vi "transform.vi"(0 "GenericTrajectory in":refnum<class "TrajectoryDL091126GenericVoxel.lvclass">, 1 "block size":i32=100000, 2 "number of pixels (all: -1)":i32=-1, 5 "transformation parameters":T1={"scale factor"=1.0, "rotation angle"=0.0, "tilting angle"=0.0, "offset"=refnum}, 11 "error in (no error)":errorcluster) -> (4 "GenericTrajectory out":refnum<class "TrajectoryDL091126GenericVoxel.lvclass">, 6 "x coordinates":dbl[unit][](array[numeric]), 8 "y coordinates":dbl[unit][](array[numeric]), 10 "z coordinates":dbl[unit][](array[numeric]), 15 "error out":errorcluster)   [LabVIEW 2010, in "TrajectoryDL091126GenericVoxel.lvclass"]
uses:
  TrajectoryDL091126GenericVoxel.lvclass
  transformation_parameters.ctl
  common/classes/SpaceVector/SpaceVector/SpaceVector.lvclass
  common/enumerations/x_y_z_enumeration.ctl
  common/enumerations/functional_global_action_enum.ctl
  TrajectoryDL091126GenericVoxel.lvclass/TrajectoryDL091126GenericVoxel.ctl
  <vilib>/Analysis/Matrix/Numeric/Conversions/Array To Matrix - RA2.vi
  <vilib>/Analysis/baseanly.llb/Real A x B.vi
  <vilib>/Analysis/Matrix/Numeric/Conversions/Matrix To Array - RM.vi
  common/classes/ErrorController/ErrorController/class_data.vi
  <vilib>/Analysis/Matrix/NI_Matrix.lvlib
  <vilib>/Analysis/NI_AALBase.lvlib
  common/classes/ErrorController/ErrorController/ErrorController.lvclass
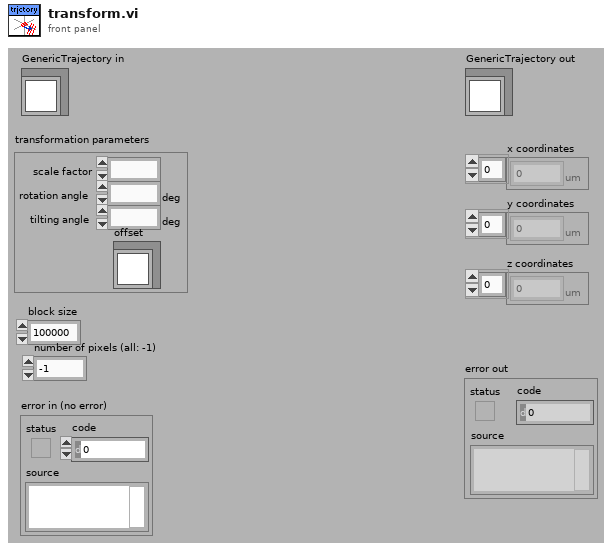
[diagram p1: front panel]
types:
  T1 = typedef "TrajectoryDL091126GenericVoxel.lvclass/transformation_parameters.ctl" = cluster{"scale factor":dbl, "rotation angle":dbl[unit], "tilting angle":dbl[unit], "offset":refnum<class "SpaceVector.lvclass">}
  T2 = typedef "x_y_z_enumeration.ctl" = enum16{"x", "y", "z"}
  T3 = typedef "functional_global_action_enum.ctl" = enum16{"get", "set", "reset"}
  T4 = typedef "NI_Matrix.lvlib/RealMatrix.ctl" = dbl[][]
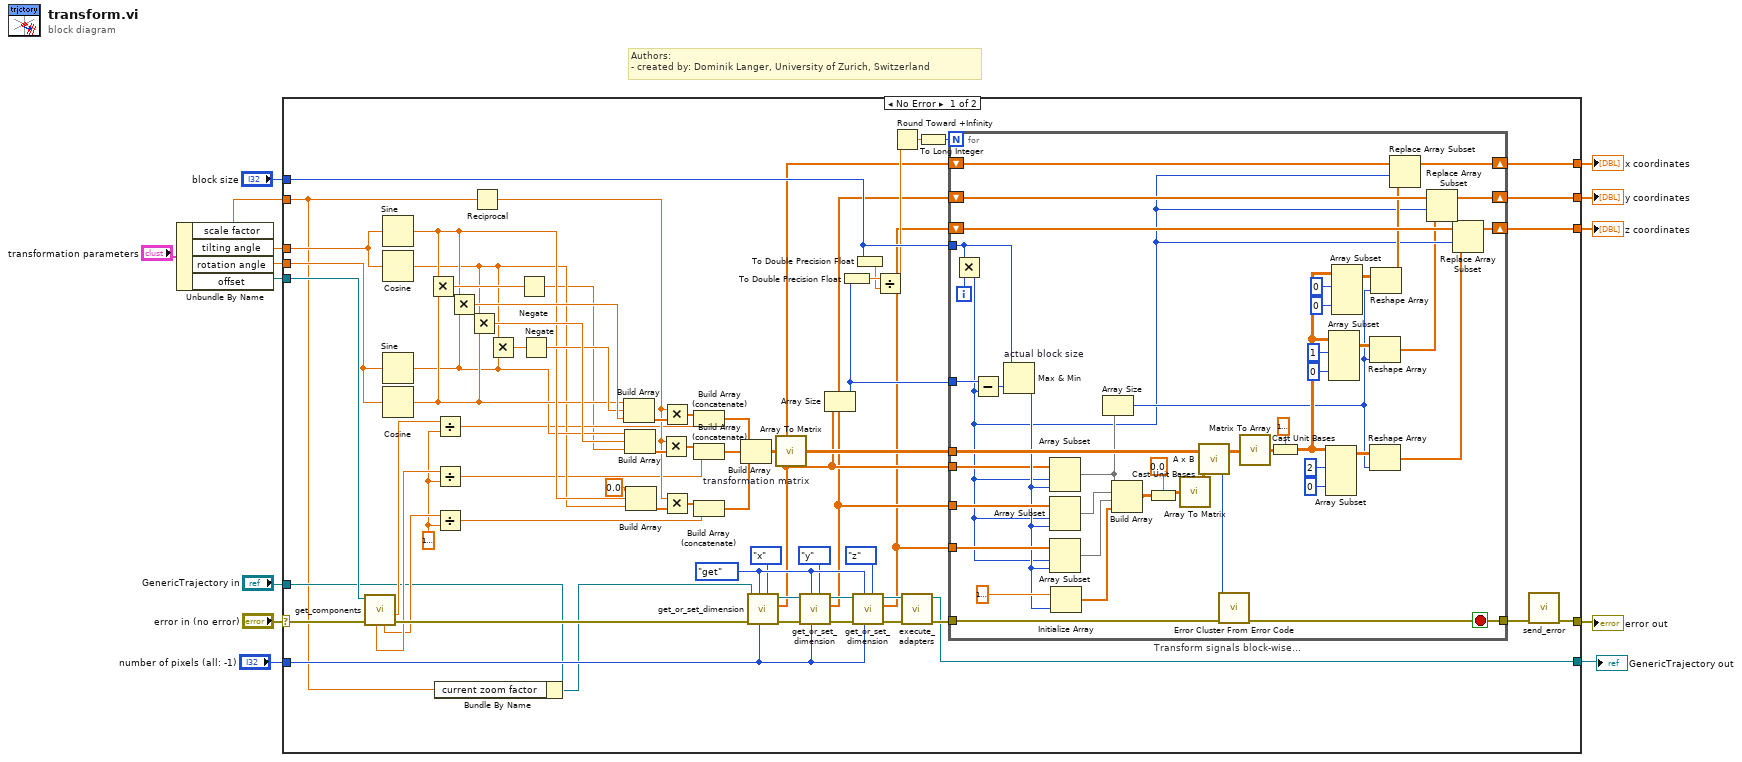
[diagram p0: block diagram]
diagram:
  # "Authors: \n- created by: Dominik Langer, University of Zurich, Switzerland"
  n1 = Unbundle By Name("transformation parameters") -> ("scale factor"=w8:dbl, "tilting angle"=w7:dbl[unit], "rotation angle"=w6:dbl[unit], "offset"=w5:refnum<class "SpaceVector.lvclass">)
  n2 = case shown="No Error" "error in (no error)" {
    selector: "error in (no error)" -> [w66 w127]
    tunnel: [w22 w127] -> w13
    tunnel: [w38 w126] -> w11
    tunnel: "GenericTrajectory in" -> [w18 w126]
    tunnel: w5 -> [w64 _]
    tunnel: w7 -> [w63 _]
    tunnel: w8 -> [w16 _]
    tunnel: "block size" -> [w51 _]
    tunnel: w6 -> [w53 _]
    tunnel: [w49 _] -> w4
    tunnel: [w48 _] -> w3
    tunnel: [w47 _] -> w2
    tunnel: "number of pixels (all: -1)" -> [w24 _]
    frame No Error {
      w34 = dbl[unit] 1e-06 ("unit (none)")
      w78 = functional_global_action_enum."get" ("action")
      n3 = call "get_components.vi"("error in (no error)"=w66, "SpaceVector in"=w64) -> ("error out"=w65:errorcluster, "x"=w37:dbl[unit], "z"=w35:dbl[unit], "y"=w36:dbl[unit])  [unwired: 4 in, 2 out]
      n4 = Sine(x=w63) -> (sin(x)=w62:dbl)
      n5 = Cosine(x=w63) -> (cos(x)=w59:dbl)
      n6 = Sine(x=w53) -> (sin(x)=w60:dbl)
      n7 = Cosine(x=w53) -> (cos(x)=w61:dbl)
      n8 = Multiply(x=w62, y=w61) -> (x*y=w71:dbl)
      n9 = Divide(x=w37, y=w34) -> (x/y=w32:dbl)
      n10 = Divide(x=w36, y=w34) -> (x/y=w28:dbl)
      n11 = Divide(x=w35, y=w34) -> (x/y=w27:dbl)
      n12 = Bundle By Name(cluster=w18, "current zoom factor"=w16) -> (w17:refnum<class "TrajectoryDL091126GenericVoxel.lvclass">)
      n13 = Multiply(x=w62, y=w60) -> (x*y=w69:dbl)
      n14 = Multiply(x=w59, y=w61) -> (x*y=w70:dbl)
      n15 = Reciprocal(x=w16) -> (1/x=w42:dbl)
      n16 = Multiply(x=w59, y=w60) -> (x*y=w67:dbl)
      n17 = Negate(x=w71) -> (-x=w15:dbl)
      n18 = Negate(x=w67) -> (-x=w68:dbl)
      n19 = Build Array(w61, w68, w69) -> (w56:dbl[])
      n20 = Build Array(w60, w70, w15) -> (w55:dbl[])
      n21 = Build Array(0.0, w62, w59) -> (w54:dbl[])
      n22 = Multiply(x=w42, y=w55) -> (x*y=w30:dbl[])
      n23 = Multiply(x=w42, y=w56) -> (x*y=w33:dbl[])
      n24 = Multiply(x=w42, y=w54) -> (x*y=w29:dbl[])
      n25 = Build Array (concatenate)(w33, w32) -> (w31:dbl[])
      n26 = Build Array (concatenate)(w30, w28) -> (w26:dbl[])
      n27 = Build Array (concatenate)(w29, w27) -> (w25:dbl[])
      n28 = Build Array "transformation matrix"(w31, w26, w25) -> (w57:dbl[][])
      n29 = call-dynamic "get_or_set_dimension.vi"("dimension"=x_y_z_enumeration."x", "number of pixels to get (-1: get all)"=w24, "action"=w78, "error in (no error)"=w65, "GenericTrajectory in"=w17) -> ("error out"=w80:errorcluster, "pixel values out (single dimension)"=w21:dbl[unit][], "GenericTrajectory out"=w74:refnum<class "TrajectoryDL091126GenericVoxel.lvclass">)  [unwired: 4 in]
      n30 = call-poly <vilib>:"Array To Matrix.vi"("Real 2D Array"=w57) -> ("Real Matrix"=w58:T4)
      n31 = call-dynamic "get_or_set_dimension.vi"("dimension"=x_y_z_enumeration."y", "number of pixels to get (-1: get all)"=w24, "action"=w78, "error in (no error)"=w80, "GenericTrajectory in"=w74) -> ("error out"=w79:errorcluster, "pixel values out (single dimension)"=w20:dbl[unit][], "GenericTrajectory out"=w73:refnum<class "TrajectoryDL091126GenericVoxel.lvclass">)  [unwired: 4 in]
      n32 = Array Size(array=w21) -> (size(s)=w46:i32)
      n33 = To Double Precision Float(number=w46) -> (double precision float=w52:dbl)
      n34 = call-dynamic "get_or_set_dimension.vi"("dimension"=x_y_z_enumeration."z", "number of pixels to get (-1: get all)"=w24, "action"=w78, "error in (no error)"=w79, "GenericTrajectory in"=w73) -> ("error out"=w41:errorcluster, "pixel values out (single dimension)"=w19:dbl[unit][], "GenericTrajectory out"=w39:refnum<class "TrajectoryDL091126GenericVoxel.lvclass">)  [unwired: 4 in]
      n35 = To Double Precision Float(number=w51) -> (double precision float=w50:dbl)
      n36 = Divide(x=w52, y=w50) -> (x/y=w45:dbl)
      n37 = Round Toward +Infinity(x=w45) -> (ceil(x): smallest int >= x=w44:dbl)
      n38 = call-dynamic "execute_adapters.vi"("error in (no error)"=w41, "GenericTrajectory in"=w39) -> ("error out"=w40:errorcluster, "GenericTrajectory out"=w38:refnum<class "TrajectoryDL091126GenericVoxel.lvclass">)  [unwired: 8 in]
      n39 = To Long Integer(number=w44) -> (32bit integer=w43:i32)
      n40 = for "Transform signals block-wise..." {
        N: w43 -> [_]
        tunnel: w20 -> [w125]
        tunnel: w19 -> [w124]
        tunnel: w58 -> [w123]
        tunnel: w21 -> [w105]
        tunnel: w51 -> [w87]
        shift-right: [w91] -> w49
        shift-left: w21 -> [w94]
        shift-right: [w90] -> w48
        shift-left: w20 -> [w93]
        shift-right: [w89] -> w47
        shift-left: w19 -> [w92]
        tunnel: w46 -> [w88]
        tunnel: w40 -> [w122]
        tunnel: [w85] -> w23
        i -> [w86]
        stop <- w85 stop-if-true
        n41 = Multiply(x=w87, y=w86) -> (x*y=w83:i32)
        n42 = Subtract(x=w88, y=w83) -> (x-y=w107:i32)
        n43 = Max & Min "actual block size"(x=w87, y=w107) -> (min(x,y)=w106:i32)  [unwired: 1 out]
        n44 = Array Subset(array=w105, index=w83, length=w106) -> (w104:dbl[unit][])
        n45 = Array Subset(array=w125, index=w83, length=w106) -> (w121:dbl[unit][])
        n46 = Array Subset(array=w124, index=w83, length=w106) -> (w120:dbl[unit][])
        n47 = Initialize Array(dbl[unit] 1e-06 ("element"), w106) -> (w112:dbl[unit][])
        n48 = Array Size(array=w104) -> (size(s)=w95:i32)
        n49 = Build Array(w104, w121, w120, w112) -> (w118:dbl[unit][][])
        n50 = Cast Unit Bases(0:w118, 1:0.0 ("unit (none)")) -> (2:w116:dbl[][])
        n51 = call-poly <vilib>:"Array To Matrix.vi"("Real 2D Array"=w116) -> ("Real Matrix"=w119:T4)
        n52 = call-poly <vilib>:"A x B.vi"("B"=w119, "A"=w123) -> ("error"=w115:i32, "A x B"=w114:T4)
        n53 = call <vilib>:"Error Cluster From Error Code.vi"("error in (no error)"=w122, "error code (0)"=w115) -> ("error out"=w85:errorcluster)  [unwired: 7 in]
        n54 = call-poly <vilib>:"Matrix To Array.vi"("Real Matrix"=w114) -> ("Real 2D Array"=w111:dbl[][])
        n55 = Cast Unit Bases(0:w111, 1:dbl[unit] 1e-06 ("element")) -> (2:w96:dbl[unit][][])
        n56 = Array Subset(array=w96, index (row)=2 ("index"), index (col)=0 ("index")) -> (w103:dbl[unit][][])  [unwired: 2 in]
        n57 = Array Subset(array=w96, index (row)=1 ("index"), index (col)=0 ("index")) -> (w97:dbl[unit][][])  [unwired: 2 in]
        n58 = Array Subset(array=w96, index (row)=0 ("index"), index (col)=0 ("index")) -> (w98:dbl[unit][][])  [unwired: 2 in]
        n59 = Reshape Array(w97, w95) -> (w82:dbl[unit][])
        n60 = Reshape Array(w103, w95) -> (w81:dbl[unit][])
        n61 = Reshape Array(w98, w95) -> (w84:dbl[unit][])
        n62 = Replace Array Subset(array=w94, new element=w84, index=w83) -> (w91:dbl[unit][])
        n63 = Replace Array Subset(array=w93, new element=w82, index=w83) -> (w90:dbl[unit][])
        n64 = Replace Array Subset(array=w92, new element=w81, index=w83) -> (w89:dbl[unit][])
      }
      n65 = call "send_error.vi"("error in (no error)"=w23) -> ("error out"=w22:errorcluster)  [unwired: 10 in]
    }
    frame Error {
    }
  }
  "error out" <- w13
  "GenericTrajectory out" <- w11
  "x coordinates" <- w4
  "y coordinates" <- w3
  "z coordinates" <- w2
